vi "start.vi"(8 "error in (no error)":errorcluster, 11 "WriteSignalsGenericPlugin in":refnum<class "SignalWriterMH110203USBStepperMotor.lvclass">) -> (0 "error out":errorcluster, 3 "WriteSignalsGenericPlugin out":refnum<class "SignalWriterMH110203USBStepperMotor.lvclass">)   [LabVIEW 2010, in "SignalWriterMH110203USBStepperMotor.lvclass"]
uses:
  SignalWriterMH110203USBStepperMotor.lvclass
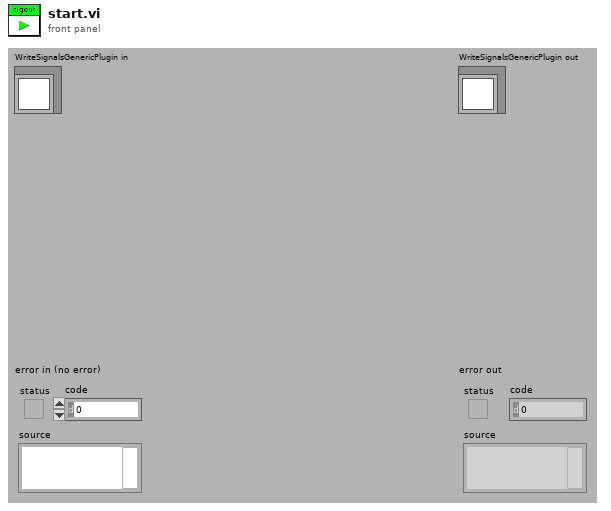
[diagram p1: front panel]
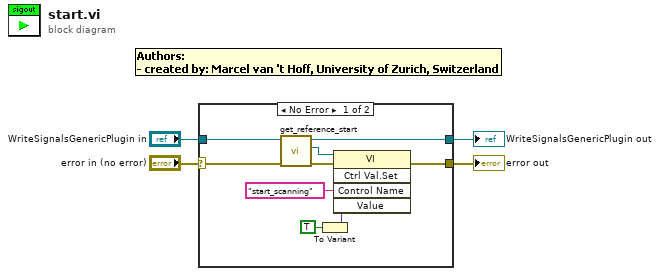
[diagram p0: block diagram]
diagram:
  n1 = case shown="No Error" "error in (no error)" {
    selector: "error in (no error)" -> [w11 w14]
    tunnel: [w13 w14] -> w2
    tunnel: [w5 w15] -> w1
    tunnel: "WriteSignalsGenericPlugin in" -> [w12 w15]
    frame No Error {
      n2 = call-dynamic "get_reference_start.vi"("error in (no error)"=w11, "SignalWriterMH110203USBStepperMotor in"=w12) -> ("error out"=w7:errorcluster, "vi reference"=w6:refnum<vi>, "SignalWriterMH110203USBStepperMotor out"=w5:refnum<class "SignalWriterMH110203USBStepperMotor.lvclass">)  [unwired: 7 in]
      n3 = To Variant(anything=TRUE) -> (Variant=w9:variant)
      n4 = invoke class="VI" method="Ctrl Val.Set"(reference=w6, error in=w7, "Control Name"="start_scanning", "Value"=w9) -> (error out=w13:errorcluster)  [unwired: 1 in, 4 out]
    }
    frame Error {
    }
  }
  "error out" <- w2
  "WriteSignalsGenericPlugin out" <- w1
